vi "fgv_ycar_arduino.vi"(7 "cmd":enum16{"init", "read", "write", "close"}(ring), 8 "error in":errorcluster, 11 "cmd":string) -> (0 "error out":errorcluster, 2 "val":bool, 3 "read_buffer":string)   [LabVIEW 2019]
uses:
  <vilib>/Instr/_visa.llb/VISA Configure Serial Port (Instr).vi
panel:
  out "cmd out":string
  out "send_data":u8[](array[numeric]) format="%x"
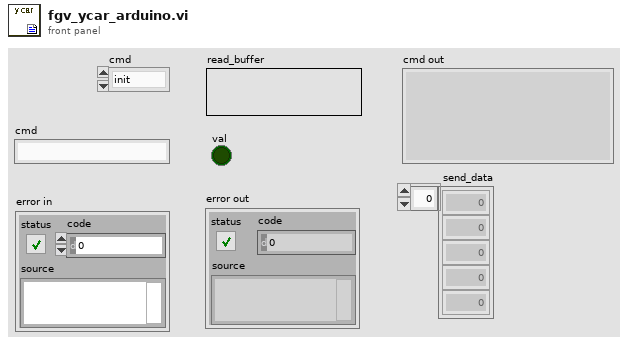
[diagram p1: front panel]
types:
  T1 = cluster{"Port":refnum<visa-resource-name>, "speed limits":cluster{"speed-limit":dbl, "steer-limit":dbl}, "limits":cluster{"speed limits":cluster{"max":dbl, "min":dbl}, "steer limits":cluster{"max":dbl, "min":dbl}}}
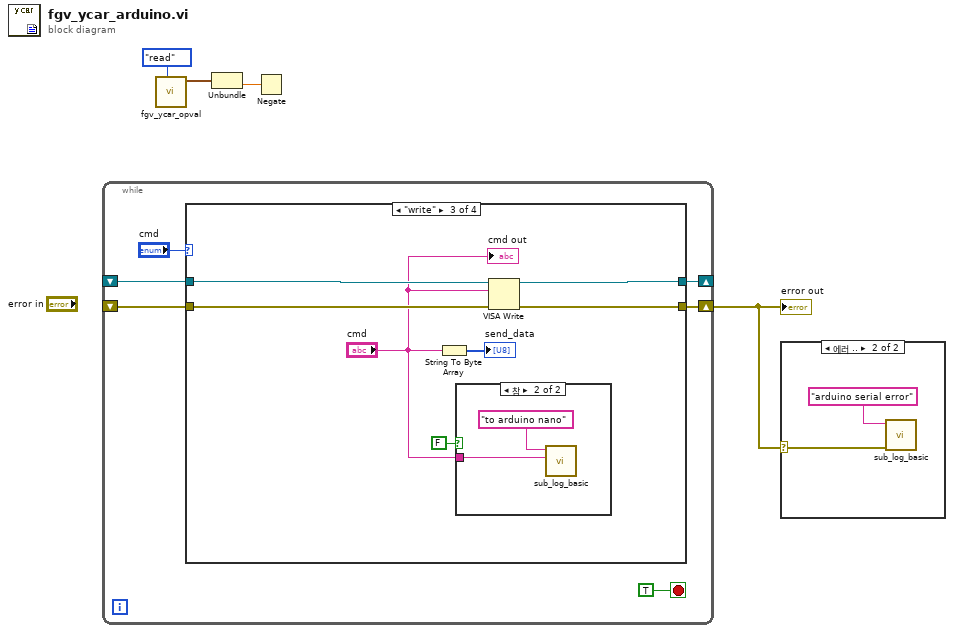
[diagram p0: block diagram]
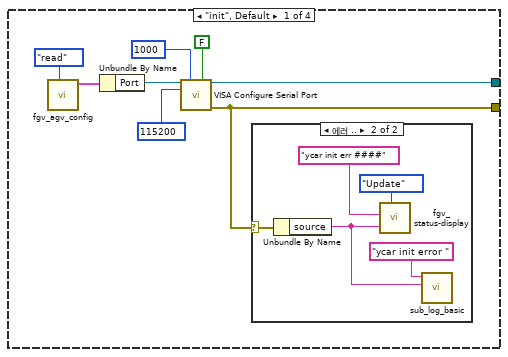
[diagram p3: hidden frame]
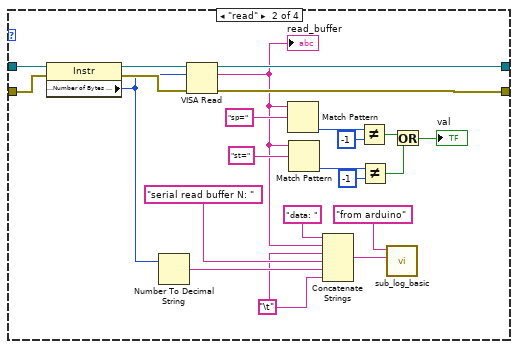
[diagram p5: hidden frame]
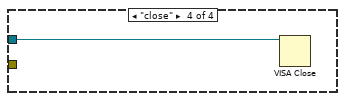
[diagram p7: hidden frame]
diagram:
  n1 = while {
    shift-right: [w8] -> _
    shift-left: _ -> [w6]
    shift-right: [w7] -> w4
    shift-left: _ -> [w5]
    stop <- TRUE stop-if-true
    n2 = case shown="\"write\"" "cmd" {
      tunnel: [w17 w44 w51 _] -> w8
      tunnel: [w11 w43 w50 _] -> w7
      tunnel: w6 -> [_ w46 w52 w56]
      tunnel: w5 -> [_ w41 w53 _]
      frame "init", Default {
        n3 = call "fgv_agv_config.vi"("cmd"=enum16{"read", "write"}."read") -> ("AGV cfg out"=w13:T1)  [unwired: 9 in, 1 out]
        n4 = Unbundle By Name(w13) -> ("Port"=w12:refnum<visa-resource-name>)
        n5 = call-poly "VISA Configure Serial Port"("VISA resource name"=w12, "timeout (10sec)"=u32 1000, "Enable Termination\nChar (T)"=FALSE ("Enable Termination\nChar (T)"), "baud rate (9600)"=u32 115200) -> ("VISA resource name out"=w17:refnum<visa-resource-name>, "error out"=w11:errorcluster)  [unwired: 10 in]
        n6 = case shown="에러 .." w11 {
          selector: w11 -> [_ w21]
          frame No Error {
          }
          frame Error {
            n7 = Unbundle By Name(w21) -> ("source"=w19:string)
            n8 = call "fgv_status-display.vi"("Mode"=enum16{"Initial", "Update", "Clear"}."Update", "detail"=w19, "title"="ycar init err ####" ("String in")) -> ()  [unwired: 8 in, 1 out]
            n9 = call "sub_log_basic.vi"("desc"=w19, "Title"="ycar init error ") -> ()  [unwired: 9 in, 1 out]
          }
        }
      }
      frame "read" {
        w26 = "\t"
        n10 = property class="Instr"(reference=w46, error in=w41) -> (reference out=w45:refnum<visa-resource-name>, error out=w42:errorcluster, "Serial Settings:Number of Bytes at Serial Port"=w30:u32)
        n11 = Number To Decimal String(number=w30) -> (decimal integer string=w28:string)  [unwired: 1 in]
        n12 = VISA Read(VISA resource name=w45, byte count=w30, error in (no error)=w42) -> (VISA resource name out=w44:refnum<visa-resource-name>, read buffer=w24:string, error out=w43:errorcluster)  [unwired: 1 out]
        "read_buffer" <- w24
        n13 = Match Pattern(string=w24, regular expression="sp=") -> (offset past match=w39:i32)  [unwired: 1 in, 3 out]
        n14 = Match Pattern(string=w24, regular expression="st=") -> (offset past match=w36:i32)  [unwired: 1 in, 3 out]
        n15 = Concatenate Strings("data: " ("문자열"), w24, w26, "serial read buffer N: " ("문자열"), w28, w26) -> (w25:string)
        n16 = Not Equal?(x=w39, y=-1) -> (x != y?=w34:bool)
        n17 = Not Equal?(x=w36, y=-1) -> (x != y?=w35:bool)
        n18 = call "sub_log_basic.vi"("desc"=w25, "Title"="from arduino") -> ()  [unwired: 9 in, 1 out]
        n19 = Or(x=w34, y=w35) -> (x .or. y?=→"val":bool)
      }
      frame "write" {
        n20 = String To Byte Array(string="cmd") -> (unsigned byte array=→"send_data":u8[])
        n21 = case shown="참" FALSE {
          tunnel: "cmd" -> [_ w54]
          frame False {
          }
          frame True {
            n22 = call "sub_log_basic.vi"("desc"=w54, "Title"="to arduino nano") -> ()  [unwired: 9 in, 1 out]
          }
        }
        n23 = VISA Write(VISA resource name=w52, write buffer="cmd", error in (no error)=w53) -> (VISA resource name out=w51:refnum<visa-resource-name>, error out=w50:errorcluster)  [unwired: 1 out]
        "cmd out" <- "cmd"
      }
      frame "close" {
        n24 = VISA Close(VISA resource name=w56) -> ()  [unwired: 1 in, 1 out]
      }
    }
  }
  "error out" <- w4
  n25 = call "fgv_ycar_opval.vi"("cmd"=enum16{"read", "write", "ini"}."read") -> ("opval out"=w2:cluster{"speed":dbl, "steer":dbl})  [unwired: 10 in]
  n26 = Unbundle(w2) -> ("steer"=w3:dbl)  [unwired: 1 out]
  n27 = Negate(x=w3) -> ()  [unwired: 1 out]
  n28 = case shown="에러 .." w4 {
    selector: w4 -> [_ w57]
    frame No Error {
    }
    frame Error {
      n29 = call "sub_log_basic.vi"("error in"=w57, "Title"="arduino serial error") -> ()  [unwired: 9 in, 1 out]
    }
  }
